vi "Set Path.vi"(10 "Path":path, 11 "Base Sender in":refnum<class "Base Sender.lvclass">) -> (3 "Base Sender out":refnum<class "Base Sender.lvclass">)   [LabVIEW 2021, in "jettl.lvlib" / "Sender.lvlib" / "Base Sender.lvclass"]
uses:
  Base Sender.lvclass
  Base Sender.lvclass/Base Sender.ctl
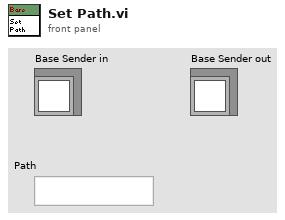
[diagram p1: front panel]
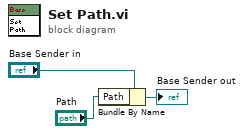
[diagram p0: block diagram]
diagram:
  n1 = Bundle By Name(cluster="Base Sender in", "Path"="Path") -> (→"Base Sender out":refnum<class "Base Sender.lvclass">)
